vi "Get Num Positions.vi"(0 "Notifier Name":string, 11 "Error In":errorcluster) -> (4 "Notifier Name Dup":string, 8 "Num Pos":i32[](array[numeric]), 15 "Error Out":errorcluster)   [LabVIEW 2020]
doc: "Array out put is as follow. 0: Number of disk positions. 1: Number of dichroic positions. 2: Number of filter wheel positions."
uses:
  Spinning Disk Type Defs/SD Notifer Data.ctl
  Spinning Disk Type Defs/SD Actions.ctl
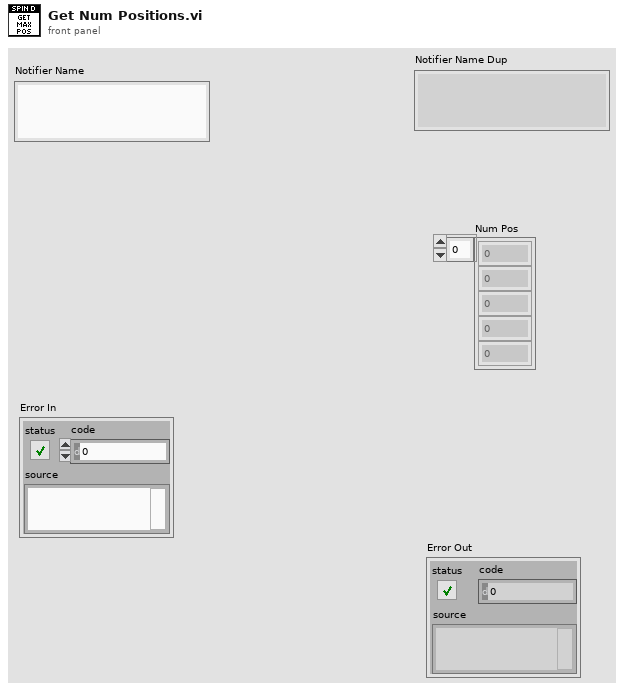
[diagram p1: front panel]
types:
  T1 = typedef "SD Notifer Data.ctl" = cluster{"Actions":T2, "Disk On?":bool, "Dichroic Pos.":i32, "Filter Wheel Pos.":i32, "Disk Pos.":i32, "Recived":bool, "Num Pos":i32[]}
  T2 = typedef "SD Actions.ctl" = enum16{"Status", "Get All Pos.", "Get Num. Pos.", "Home All", "Set Filter Wheel Pos.", "Set Disk Pos.", "Set Dichroic Pos.", "Disk On", "Disk Off", "Quit"}
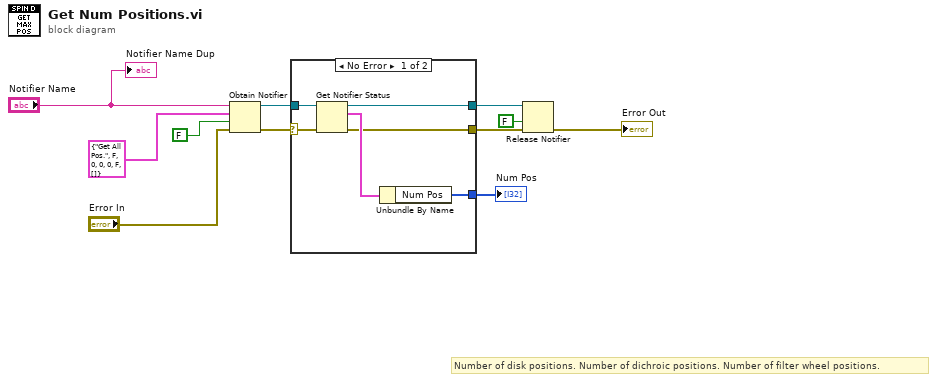
[diagram p0: block diagram]
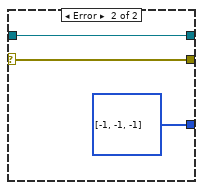
[diagram p2: hidden frame]
diagram:
  # "Number of disk positions. Number of dichroic positions. Number of filter wheel positions."
  n1 = Obtain Notifier(name (unnamed)="Notifier Name", notification data type=T1 {"Actions"=enum."Get All Pos.", "Disk On?"=FALSE, "Dichroic Pos."=0, "Filter Wheel Pos."=0, "Disk Pos."=0, "Recived"=FALSE, "Num Pos"=[]} ("XLight Notifier Data"), create if not found? (T)=FALSE, error in (no error)="Error In") -> (notifier out=w7:refnum<notifier>, error out=w4:errorcluster)  [unwired: 1 out]
  n2 = case shown="No Error" w4 {
    selector: w4 -> [w14 w19]
    tunnel: w7 -> [w17 w20]
    tunnel: [w16 w20] -> w6
    tunnel: [w13 w19] -> w3
    tunnel: [w12 i32[] [-1, -1, -1] ("Num Pos")] -> w1
    frame No Error {
      n3 = Get Notifier Status(notifier=w17, error in (no error)=w14) -> (notifier out=w16:refnum<notifier>, current notification=w15:T1, error out=w13:errorcluster)  [unwired: 2 out]
      n4 = Unbundle By Name(w15) -> ("Num Pos"=w12:i32[])
    }
    frame Error {
    }
  }
  "Num Pos" <- w1
  n5 = Release Notifier(notifier=w6, force destroy? (F)=FALSE, error in (no error)=w3) -> (error out=→"Error Out":errorcluster)  [unwired: 2 out]
  "Notifier Name Dup" <- "Notifier Name"
